vi "Stop Target Refresh.vi"(8 "Error In":errorcluster) -> (0 "Error Out":errorcluster)   [LabVIEW 2019, in "Project.Dependencies Finder.lvlib"]
doc: "Abort any active target refresh and stops the Target Refresh Tracker.\n\n2020-12-07: Henrik Dueholm Hansen"
uses:
  Project.Dependencies Finder.lvlib
  Private/Gobal_Progress Tracking State.vi
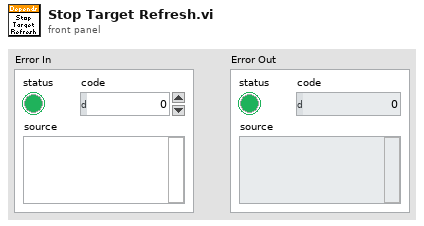
[diagram p1: front panel]
types:
  T1 = typedef "Project.Dependencies Finder.lvlib/Ctl_Progress Queue.ctl" = refnum<queue>
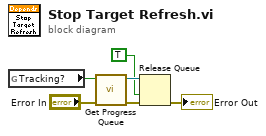
[diagram p0: block diagram]
diagram:
  n1 = global read "Gobal_Progress Tracking State.vi" "Tracking?"() -> (w1:bool)
  n2 = call "Get Progress Queue.vi"("error in"="Error In", "Enable Tracking?"=w1) -> ("error out"=w2:errorcluster, "Progress queue"=w4:T1)  [unwired: 8 in]
  n3 = Release Queue(queue=w4, force destroy? (F)=TRUE, error in (no error)=w2) -> (error out=→"Error Out":errorcluster)  [unwired: 2 out]
